vi "GetActualDepsListPath.vi"(8 "error in (no error)":errorcluster) -> (0 "error out":errorcluster, 3 "ActualDepsListPath":path)   [LabVIEW 2023, in "CICD.lvlib"]
uses:
  CICD.lvlib
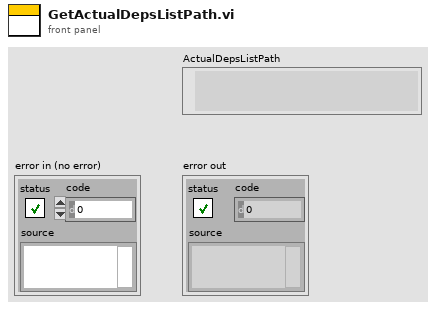
[diagram p1: front panel]
types:
  T1 = typedef "CICD.lvlib/CICDPathConfigs.ctl" = cluster{"GlobalIncludePaths":path[], "GlobalExcludePaths":path[], "BuildSpecsIncludePaths":path[], "ActualDepsIncludePaths":path[], "WorkspacePath":path, "SourceFolderPaths":path[], "ChangedFilesLogpaths":map{string, path}}
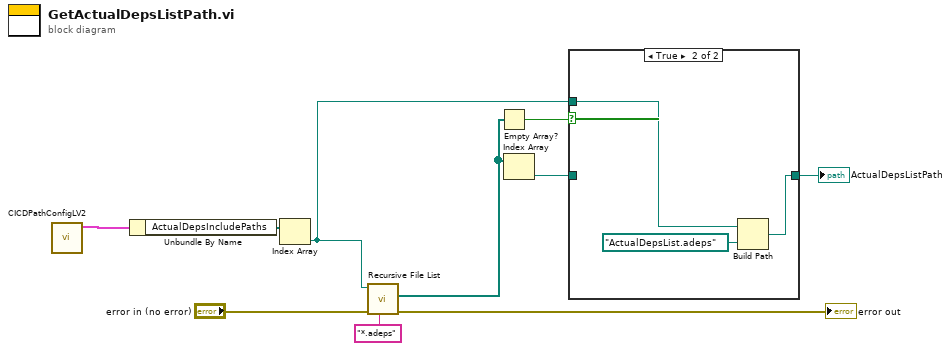
[diagram p0: block diagram]
diagram:
  n1 = call "CICDPathConfigLV2.vi"() -> ("CICD Path Config Out"=w8:T1)  [unwired: 11 in]
  n2 = Unbundle By Name(w8) -> ("ActualDepsIncludePaths"=w9:path[])
  n3 = Index Array(array=w9) -> (element=w5:path)  [unwired: 1 in]
  n4 = call <vilib>:"Recursive File List.vi"("pattern"="*.adeps", "error in (no error)"="error in (no error)", "Folder Path"=w5) -> ("error out"=→"error out":errorcluster, "All Files in Dir"=w7:path[])  [unwired: 4 in, 3 out]
  n5 = Empty Array?(array=w7) -> (empty?=w6:bool)
  n6 = Index Array(array=w7) -> (element=w4:path)  [unwired: 1 in]
  n7 = case shown="True" w6 {
    tunnel: w5 -> [_ w14]
    tunnel: w4 -> [w11 _]
    tunnel: [w11 w12] -> w3
    frame False {
    }
    frame True {
      n8 = Build Path(base path=w14, name or relative path=path "ActualDepsList.adeps") -> (appended path=w12:path)
    }
  }
  "ActualDepsListPath" <- w3
